vi "Data Read.vi"(6 "Append Index":i32 min=-1, 8 "error in (no error)":errorcluster, 11 "path":path) -> (0 "error out":errorcluster, 1 "Notes":string, 2 "Data (Dictionary)":T1[](array[typedef]), 3 "path out":path)   [LabVIEW 2019, in "Data.lvclass"]
uses:
  Data.lvclass
  Typedefs/Operation--enum.ctl
  Typedefs/File Type--enum.ctl
  Typedefs/Dictionary--cluster.ctl
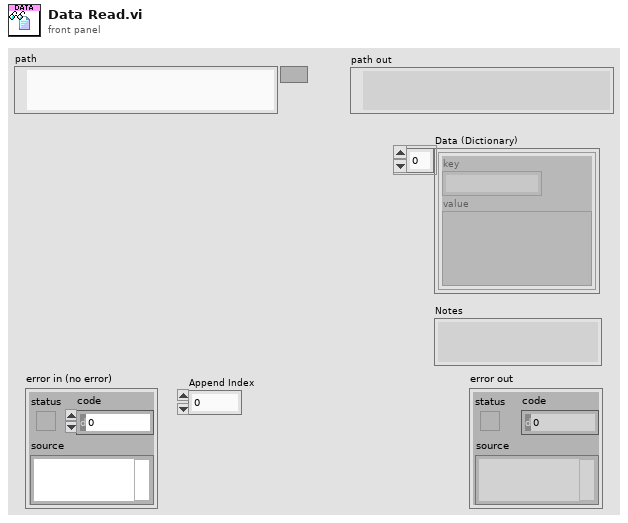
[diagram p1: front panel]
types:
  T1 = typedef "Data.lvclass/Dictionary--cluster.ctl" = cluster{"key":string, "value":variant}
  T2 = typedef "Data.lvclass/Operation--enum.ctl" = enum16{"Read", "Write", "Write + Append"}
  T3 = typedef "Data.lvclass/File Type--enum.ctl" = enum16{"DAT", "ITX", "TDMS", "VI"}
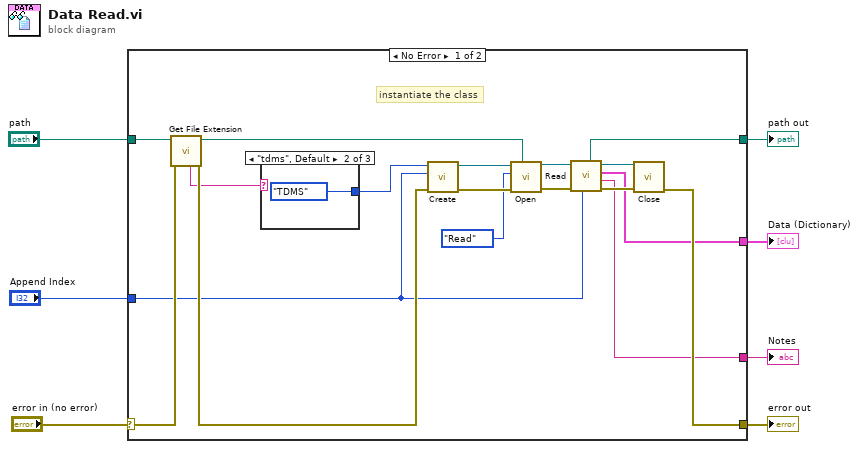
[diagram p0: block diagram]
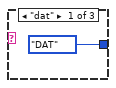
[diagram p2: hidden frame]
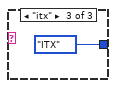
[diagram p3: hidden frame]
diagram:
  n1 = case shown="No Error" "error in (no error)" {
    selector: "error in (no error)" -> [w14 w30]
    tunnel: [w18 w30] -> w6
    tunnel: [w17 w29] -> w5
    tunnel: "path" -> [w12 w29]
    tunnel: [w16 _] -> w2
    tunnel: [w15 _] -> w3
    tunnel: "Append Index" -> [w8 _]
    frame No Error {
      # "instantiate the class"
      n2 = call <vilib>:"Get File Extension.vi"("error in (no error)"=w14, "file"=w12) -> ("error out"=w13:errorcluster, "dup file"=w11:path, "unmodified file extension"=w10:string)  [unwired: 5 in, 2 out]
      n3 = case shown="\"tdms\", Default" w10 {
        tunnel: [File_Type--enum."DAT" ("File Type") File_Type--enum."TDMS" ("File Type") File_Type--enum."ITX" ("File Type")] -> w9
        frame "dat" {
        }
        frame "tdms", Default {
        }
        frame "itx" {
        }
      }
      n4 = call "Create.vi"("error in (no error)"=w13, "Append Index (-1)"=w8, "File Type"=w9) -> ("error out"=w24:errorcluster, "Data out"=w25:refnum<class "Data.lvclass">)  [unwired: 7 in]
      n5 = call-dynamic "Open.vi"("Path"=w11, "error in (no error)"=w24, "Operation"=Operation--enum."Read", "Data in"=w25) -> ("error out"=w22:errorcluster, "Data out"=w23:refnum<class "Data.lvclass">)  [unwired: 6 in]
      n6 = call-dynamic "Read.vi"("Append Index"=w8, "error in (no error)"=w22, "Data Save in"=w23) -> ("error out"=w20:errorcluster, "Notes"=w15:string, "Data (Dictionary)"=w16:T1[], "Data Save out"=w19:refnum<class "Data.lvclass">, "Path out"=w17:path)  [unwired: 4 in]
      n7 = call-dynamic "Close.vi"("error in (no error)"=w20, "Data in"=w19) -> ("error out"=w18:errorcluster)  [unwired: 8 in, 1 out]
    }
    frame Error {
    }
  }
  "error out" <- w6
  "path out" <- w5
  "Data (Dictionary)" <- w2
  "Notes" <- w3
